vi "EncoderClimb.vi"(6 "Zero":bool, 7 "Update":bool) -> (3 "Position_out":i32)   [LabVIEW 2015]
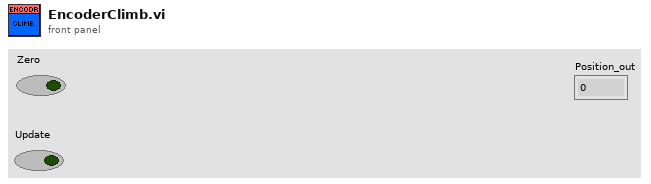
[diagram p1: front panel]
types:
  T1 = typedef "WPI_EncoderDevRef.ctl" = cluster{"DevStatus":errorcluster, "EncoderIndex":T2, "CounterIndex":T3, "DistancePerCount":dbl, "Decoding Type":T4}
  T2 = typedef "FPGA_EncoderIdx.ctl" = enum8{"Enc 0", "Enc 1", "Enc 2", "Enc 3", "Enc 4", "Enc 5", "Enc 6", "Enc 7", "Invalid"}
  T3 = typedef "FPGA_CounterCtrSystemIndex.ctl" = enum8{"Ctr 0", "Ctr 1", "Ctr 2", "Ctr 3", "Ctr 4", "Ctr 5", "Ctr 6", "Ctr 7", "Invalid"}
  T4 = typedef "WPI_EncoderType.ctl" = enum16{"1x", "2x", "4x"}
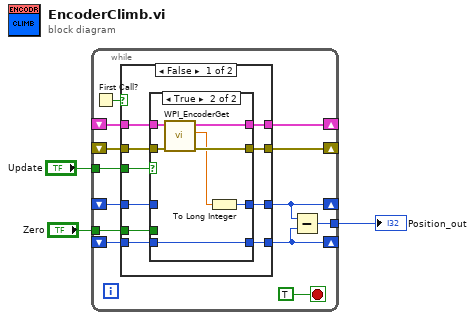
[diagram p0: block diagram]
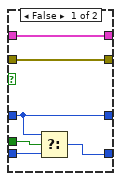
[diagram p2: hidden frame]
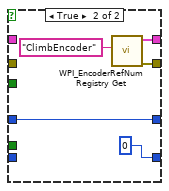
[diagram p3: hidden frame]
diagram:
  n1 = while {
    shift-right: [w4] -> _
    shift-left: _ -> [w16]
    tunnel: "Update" -> [w15]
    shift-right: [w11] -> _
    shift-left: _ -> [w12]
    tunnel: "Zero" -> [w13]
    tunnel: [w10] -> w1
    shift-right: [w7] -> _
    shift-left: _ -> [w5]
    shift-right: [w8] -> _
    shift-left: _ -> [w6]
    stop <- TRUE stop-if-true
    n2 = First Call?() -> (First Call?: T/F=w9:bool)
    n3 = case shown="False" w9 {
      tunnel: w16 -> [w26 w40]
      tunnel: w15 -> [w25 _]
      tunnel: w13 -> [w24 _]
      tunnel: w12 -> [w23 _]
      tunnel: [w22 0 ("Distance")] -> w11
      tunnel: [w19 w43] -> w8
      tunnel: [w18 w42] -> w7
      tunnel: w6 -> [w21 _]
      tunnel: w5 -> [w20 _]
      tunnel: [w17 w40] -> w4
      frame False {
        n4 = case shown="True" w25 {
          tunnel: w26 -> [w27 _]
          tunnel: w24 -> [w32 _]
          tunnel: w23 -> [w31 w39]
          tunnel: [w30 w39] -> w22
          tunnel: w21 -> [w29 w38]
          tunnel: w20 -> [w28 w37]
          tunnel: [w29 w36] -> w19
          tunnel: [w28 w35] -> w18
          tunnel: [w27 w33] -> w17
          frame False {
            n5 = Select(t=w27, s=w32, f=w31) -> (s? t:f=w30:i32)
          }
          frame True {
            n6 = call <vilib>:"WPI_EncoderGet.vi"("error in (no error)"=w37, "EncoderDevRef"=w38) -> ("error out"=w35:errorcluster, "Distance"=w34:dbl, "EncoderDevRef"=w36:T1)  [unwired: 4 in, 3 out]
            n7 = To Long Integer(number=w34) -> (32bit integer=w33:i32)
          }
        }
      }
      frame True {
        n8 = call <vilib>:"WPI_EncoderRefNum Registry Get.vi"("refnum name"="ClimbEncoder") -> ("error out"=w42:errorcluster, "EncoderDevRef"=w43:T1)  [unwired: 9 in]
      }
    }
    n9 = Subtract(x=w4, y=w11) -> (x-y=w10:i32)
  }
  "Position_out" <- w1
